vi "Ctor.vi"(8 "error in (no error)":errorcluster, 11 "Panel in":refnum<class "Panel.lvclass">) -> (0 "error out":errorcluster, 3 "Panel out":refnum<class "Panel.lvclass">)   [LabVIEW 2020, in "OOPanel.lvlib" / "Panel.lvclass"]
uses:
  Panel.lvclass
  Visibility State.ctl
  OOPanel.lvlib
  Ref Data.ctl
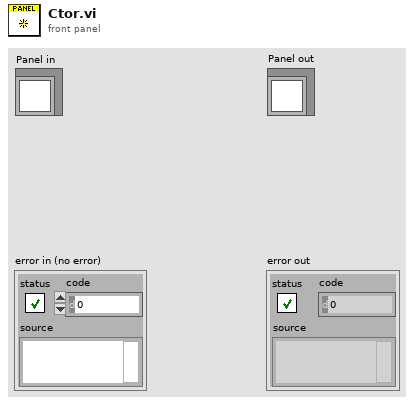
[diagram p1: front panel]
types:
  T1 = typedef "OOPanel.lvlib/Panel.lvclass/Ref Data.ctl" = cluster{"Panel Ref":refnum<vi>, "SubPanel":refnum<vi>, "Close":bool, "Running":bool, "State":T2}
  T2 = typedef "OOPanel.lvlib/Visibility State.ctl" = enum16{"Idle", "Closed", "Hidden", "Visible", "Subpanel", "Hidden Subpanel"}
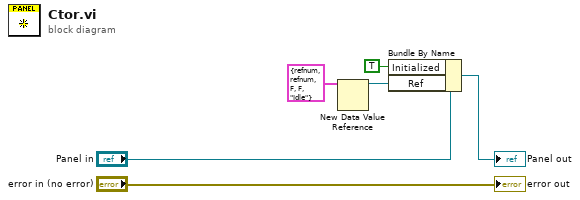
[diagram p0: block diagram]
diagram:
  n1 = New Data Value Reference(data value=T1 {"Panel Ref"=refnum, "SubPanel"=refnum, "Close"=FALSE, "Running"=FALSE, "State"=enum."Idle"} ("Ref Data")) -> (data value reference=w1:refnum<data-value>)  [unwired: 1 in, 1 out]
  n2 = Bundle By Name(cluster="Panel in", "Initialized"=TRUE, "Ref"=w1) -> (→"Panel out":refnum<class "Panel.lvclass">)
  "error out" <- "error in (no error)"
